vi "Get Subpanels to Launch.vi"(4 "Error In":errorcluster) -> (0 "Error Out":errorcluster, 3 "Subpanels to Launch":T1[](array[typedef]))   [LabVIEW 2020, in "Config Data.lvlib" / "Config Data.lvclass"]
uses:
  Config Data.lvclass
  Config Data.lvclass/Config Data.ctl
  typedefs/Launch Location.ctl
  typedefs/Process Type.ctl
  typedefs/Process Launch Data.ctl
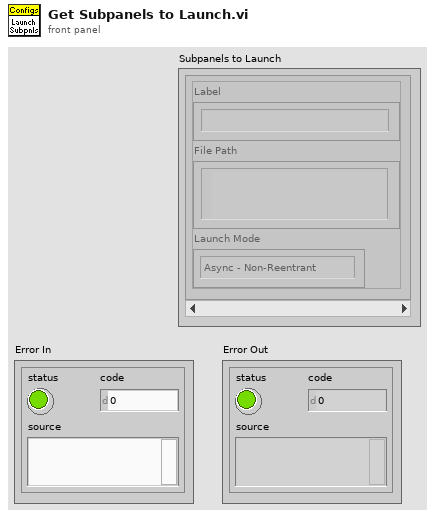
[diagram p1: front panel]
types:
  T1 = typedef "Config Data.lvlib/Config Data.lvclass/Process Launch Data.ctl" = cluster{"Label":string, "File Path":path, "Launch Mode":T2}
  T2 = typedef "Config Data.lvlib/Config Data.lvclass/Process Type.ctl" = enum16{"Async - Non-Reentrant", "Async - Reentrant", "Run Method - Non-Reentrant", "Run Method - Reentrant"}
  T3 = typedef "Config Data.lvlib/Config Data.lvclass/Launch Location.ctl" = enum16{"Startup", "Subpanels"}
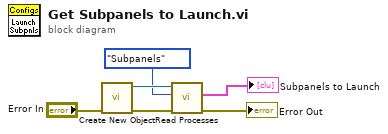
[diagram p0: block diagram]
diagram:
  n1 = call "Create New Object.vi"("Error In"="Error In") -> ("Error Out"=w5:errorcluster, "Config Data"=w4:refnum<class "Config Data.lvclass">)  [unwired: 5 in]
  n2 = call-dynamic "Read Processes.vi"("Error In"=w5, "Launch Condition"=Launch_Location."Subpanels", "Config Data in"=w4) -> ("Error Out"=→"Error Out":errorcluster, "Processes to Launch"=→"Subpanels to Launch":T1[])  [unwired: 2 in, 1 out]
